vi "myRIO v1.0 Build MUX Configuration DO Block.vi"(11 "DO (N Samples) Channel List":T4) -> (3 "Channel Reservation List":T1)   [LabVIEW 2021]
uses:
  <vilib>/myRIO/Common/Instrument Driver Framework/myRIO v1.0/DO Block/typedefs/DO Block Channels List.ctl
  <vilib>/myRIO/Common/Instrument Driver Framework/myRIO v1.0/DO Block/typedefs/DO Block Channels Enum.ctl
  <vilib>/myRIO/Common/Instrument Driver Framework/myRIO v1.0/Resource Manager/typedefs/myRIO v1.0 Channel Reservation List.ctl
  <vilib>/myRIO/Common/Instrument Driver Framework/myRIO v1.0/Resource Manager/typedefs/myRIO v1.0 Channel Reservation Info.ctl
  <vilib>/myRIO/Common/Instrument Driver Framework/myRIO v1.0/Resource Manager/typedefs/myRIO v1.0 Connector List.ctl
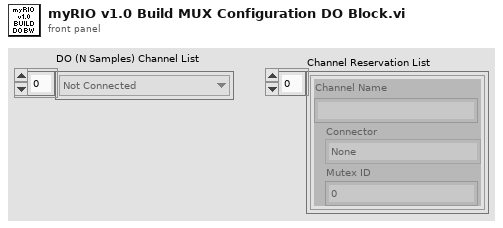
[diagram p1: front panel]
types:
  T1 = typedef "myRIO v1.0 Channel Reservation List.ctl" = T2[]
  T2 = typedef "myRIO v1.0 Channel Reservation Info.ctl" = cluster{"Channel Name":string, "Connector":T3, "Mutex ID":i32}
  T3 = typedef "myRIO v1.0 Connector List.ctl" = enum32{"None", "ConnectorA", "ConnectorB", "ConnectorC"}
  T4 = typedef "DO Block Channels List.ctl" = T5[]
  T5 = typedef "DO Block Channels Enum.ctl" = enum16{"Not Connected", "A/DO0 (N Samples)", "A/DO1 (N Samples)", "A/DO2 (N Samples)", "A/DO3 (N Samples)", "A/DO4 (N Samples)", "A/DO5 (N Samples)", "A/DO6 (N Samples)", "A/DO7 (N Samples)", "A/DO8 (N Samples)", "A/DO9 (N Samples)", "A/DO10 (N Samples)", "A/DO11 (N Samples)", "A/DO12 (N Samples)", "A/DO13 (N Samples)", "A/DO14 (N Samples)", "A/DO15 (N Samples)", "A/DO16 (N Samples)", "A/DO17 (N Samples)", "A/DO18 (N Samples)", "A/DO19 (N Samples)", "B/DO0 (N Samples)", "B/DO1 (N Samples)", "B/DO2 (N Samples)", "B/DO3 (N Samples)", "B/DO4 (N Samples)", "B/DO5 (N Samples)", "B/DO6 (N Samples)", "B/DO7 (N Samples)", "B/DO8 (N Samples)", "B/DO9 (N Samples)", "B/DO10 (N Samples)", "B/DO11 (N Samples)", "B/DO12 (N Samples)", "B/DO13 (N Samples)", "B/DO14 (N Samples)", "B/DO15 (N Samples)", "B/DO16 (N Samples)", "B/DO17 (N Samples)", "B/DO18 (N Samples)", "B/DO19 (N Samples)"}
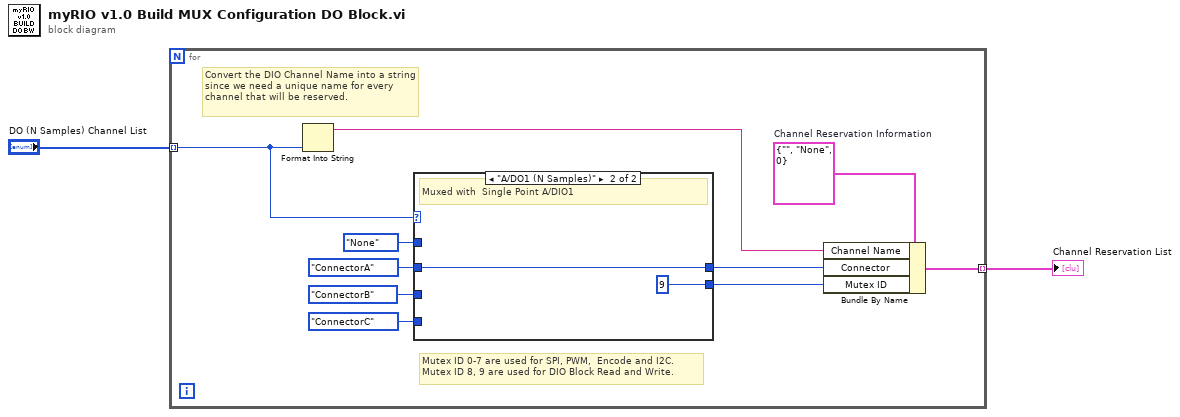
[diagram p0: block diagram]
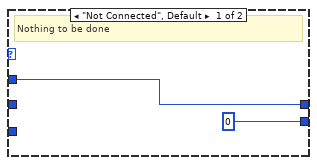
[diagram p2: hidden frame]
diagram:
  n1 = for {
    tunnel: "DO (N Samples) Channel List" -> [w6] mode=indexing
    tunnel: [w7] -> w1 mode=indexing
    w10 = T2 {"Channel Name"="", "Connector"=enum."None", "Mutex ID"=0}  # Channel Reservation Information
    # "Mutex ID 0-7 are used for SPI, PWM,  Encode and I2C.\nMutex ID 8, 9 are used for DIO Block Read and Write."
    # "Convert the DIO Channel Name into a string since we need a unique name for every channel that will be reserved."
    n2 = Format Into String(w6) -> (resulting string=w5:string)  [unwired: 3 in, 1 out]
    n3 = case shown="\"A/DO1 (N Samples)\"" w6 {
      tunnel: myRIO_v1.0_Connector_List."None" ("Connector List") -> [w14 _]
      tunnel: myRIO_v1.0_Connector_List."ConnectorA" ("Connector List") -> [_ w15]
      tunnel: [0 ("index") 9 ("index")] -> w8
      tunnel: [w14 w15] -> w9
      tunnel: myRIO_v1.0_Connector_List."ConnectorB" ("Connector List") -> [_ _]
      tunnel: myRIO_v1.0_Connector_List."ConnectorC" ("Connector List") -> [_ _]
      frame "Not Connected", Default {
        # "Nothing to be done"
      }
      frame "A/DO1 (N Samples)" {
        # "Muxed with  Single Point A/DIO1"
      }
    }
    n4 = Bundle By Name(cluster=w10, "Channel Name"=w5, "Connector"=w9, "Mutex ID"=w8) -> (w7:T2)
  }
  "Channel Reservation List" <- w1
